vi "Draw Icon.vi"(5 "Title":string, 7 "Frame Border":T2={"left"=0, "top"=0, "right"=150, "bottom"=100}, 10 "Icon Pixmap":T1, 11 "Picture In":picture) -> (3 "Picture":picture)   [LabVIEW 2022 SP3, in "FlexBlocks Support.lvlib"]
uses:
  FlexBlocks Support.lvlib
  <vilib>/picture/picture.llb/imagedata.ctl
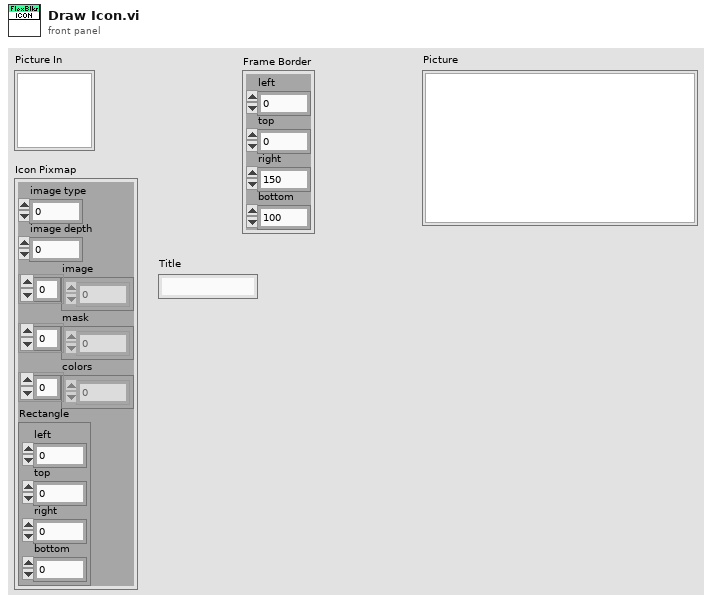
[diagram p1: front panel]
types:
  T1 = typedef "imagedata.ctl" = cluster{"image type":i32, "image depth":i32, "image":u8[], "mask":u8[], "colors":u32[], "Rectangle":cluster{"left":i16, "top":i16, "right":i16, "bottom":i16}}
  T2 = cluster{"left":i16, "top":i16, "right":i16, "bottom":i16}
  T3 = cluster{"horizontal":enum16{"left", "center", "right"}, "vertical":enum16{"top", "center", "bottom"}}
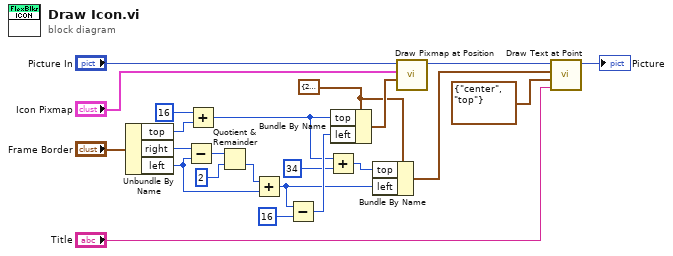
[diagram p0: block diagram]
diagram:
  w4 = cluster{"left":i16, "top":i16} {"left"=290, "top"=190} ("Position")
  n1 = Unbundle By Name("Frame Border") -> ("top"=w14:i16, "right"=w20:i16, "left"=w16:i16)
  n2 = Subtract(x=w20, y=w16) -> (x-y=w19:i16)
  n3 = Add(x=i16 16, y=w14) -> (x+y=w7:i16)
  n4 = Quotient & Remainder(x=w19, y=i16 2) -> (floor(x/y)=w17:i16)  [unwired: 1 out]
  n5 = Add(x=w17, y=w16) -> (x+y=w9:i16)
  n6 = Subtract(x=w9, y=i16 16) -> (x-y=w11:i16)
  n7 = Add(x=w7, y=i16 34) -> (x+y=w6:i16)
  n8 = Bundle By Name(cluster=w4, "top"=w7, "left"=w11) -> (w15:cluster{"left":i16, "top":i16})
  n9 = Bundle By Name(cluster=w4, "top"=w6, "left"=w9) -> (w5:cluster{"left":i16, "top":i16})
  n10 = call "Draw Pixmap at Position.vi"("Position"=w15, "Pixmap"="Icon Pixmap", "2D Picture In"="Picture In") -> ("2D Picture"=w10:picture)  [unwired: 8 in]
  n11 = call <vilib>:"Draw Text at Point.vi"("text"="Title", "alignment(left, top)"=T3 {"horizontal"=enum."center", "vertical"=enum."top"}, "origin"=w5, "picture"=w10) -> ("new picture"=→"Picture":picture)  [unwired: 6 in, 1 out]
